vi "Int 1D To Mono-Item.vi"(10 "Int Array":u32[](array[numeric])) -> (2 "Item Text":string[](array[string]))   [LabVIEW 2024]
uses:
  Int Complex To Items.vi
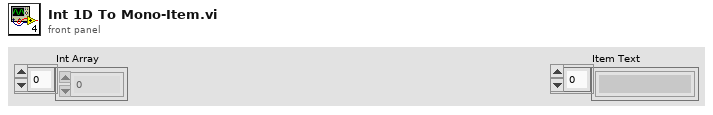
[diagram p1: front panel]
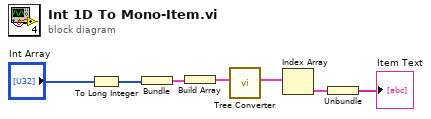
[diagram p0: block diagram]
diagram:
  n1 = To Long Integer(number="Int Array") -> (32bit integer=w5:i32[])
  n2 = Bundle(w5) -> (w7:cluster{i32[]})  [unwired: 1 in]
  n3 = Build Array(w7) -> (w6:cluster{i32[]}[])
  n4 = call-poly "Tree Converter.vi"("Numeric Array"=w6) -> ("Items Text"=w4:cluster{string[]}[])  [unwired: 10 in]
  n5 = Index Array(array=w4) -> (element=w3:cluster{string[]})  [unwired: 1 in]
  n6 = Unbundle(w3) -> (→"Item Text":string[])
